vi "SLSC Convert EDS Property to SLSC Channel Path.vi"(0 "property":T3, 1 "GUID Get Properties Page":string, 2 "GUID Set Properties Page":string, 5 "Physical Channel":string, 12 "enums":T2[](array[typedef])) -> (3 "GUID Properties Page":string, 4 "name":string, 6 "Channel out":T4, 8 "SLSC Channel Path":string="Bool.LED1.NI.GreenBool", 10 "documentation-en":string, 13 "Cluster":T1, 14 "description-en":string)   [LabVIEW 2020, in "SLSC CD System Explorer.lvlib"]
uses:
  SLSC CD API/SLSC CD System Explorer/SLSC CD System Explorer.lvlib
  <vilib>/NI VeriStand/Custom Device API/Custom Device Channel.ctl
  <vilib>/NI VeriStand/Custom Device API/Custom Device Channel Type.ctl
  JSON parsing/property.ctl
  JSON parsing/enum.ctl
  <vilib>/NI VeriStand/Custom Device API/Custom Device API.lvlib
  SLSC CD API/SLSC CD Shared/SLSC CD Shared.lvlib
  SLSC UI API/SLSC Tree Control.lvlib
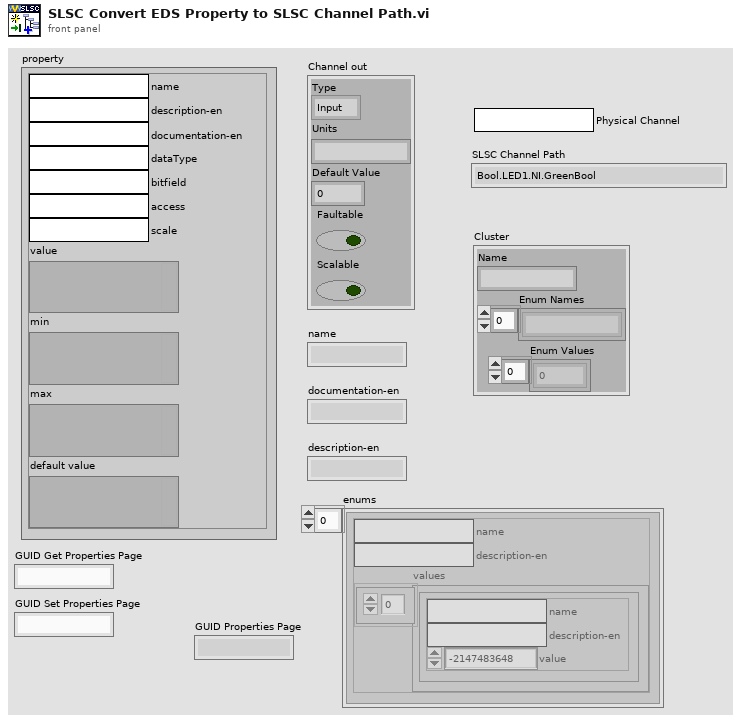
[diagram p1: front panel]
types:
  T1 = cluster{"Name":string, "Enum Names":string[], "Enum Values":i32[]}
  T2 = typedef "enum.ctl" = cluster{"name":string, "description-en":string, "values":cluster{"name":string, "description-en":string, "value":i32}[]}
  T3 = typedef "property.ctl" = cluster{"name":string, "description-en":string, "documentation-en":string, "dataType":string, "bitfield":string, "access":string, "scale":string, "value":variant, "min":variant, "max":variant, "default value":variant}
  T4 = typedef "Custom Device API.lvlib/Custom Device Channel.ctl" = cluster{"Type":T5, "Units":string, "Default Value":dbl, "Faultable":bool, "Scalable":bool}
  T5 = typedef "Custom Device API.lvlib/Custom Device Channel Type.ctl" = enum16{"Input", "Output"}
  T6 = cluster{"Name":string, "Enum Names":string[], "Enum Values":i32[]}[]
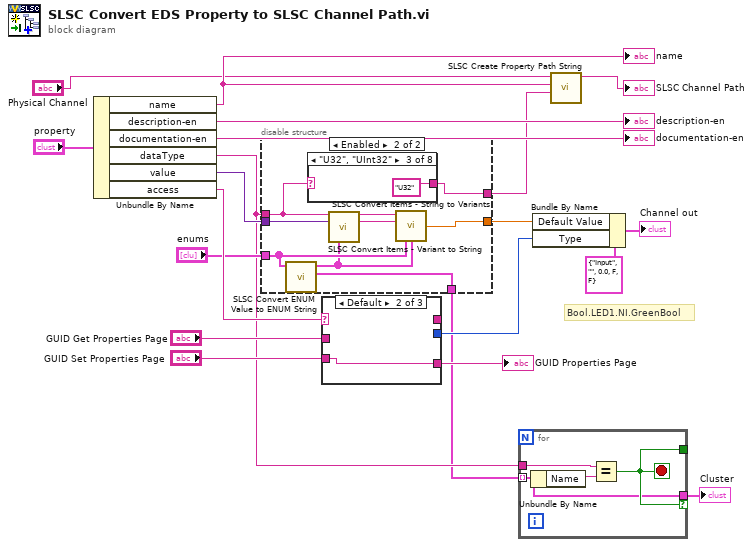
[diagram p0: block diagram]
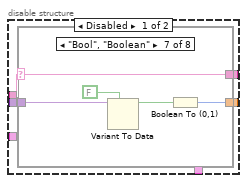
[diagram p2: hidden frame]
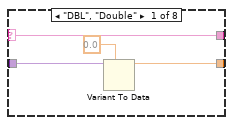
[diagram p3: hidden frame]
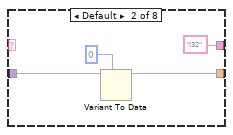
[diagram p4: hidden frame]
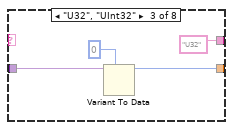
[diagram p5: hidden frame]
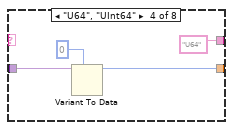
[diagram p6: hidden frame]
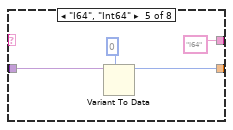
[diagram p7: hidden frame]
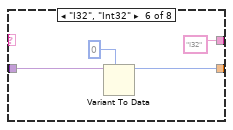
[diagram p8: hidden frame]
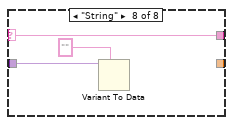
[diagram p9: hidden frame]
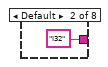
[diagram p11: hidden frame]
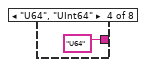
[diagram p12: hidden frame]
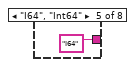
[diagram p13: hidden frame]
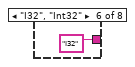
[diagram p14: hidden frame]
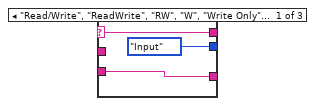
[diagram p17: hidden frame]
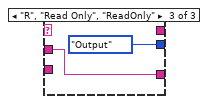
[diagram p18: hidden frame]
diagram:
  # "Bool.LED1.NI.GreenBool"
  n1 = Unbundle By Name("property") -> ("name"=w13:string, "description-en"=→"description-en":string, "documentation-en"=→"documentation-en":string, "dataType"=w3:string, "value"=w15:variant, "access"=w8:string)
  "name" <- w13
  n2 = disable-structure shown="Enabled" {
    disable-tunnel: w3 -> [w24 w59]
    disable-tunnel: w15 -> [w23 w63]
    disable-tunnel: [w22 w62] -> w14
    disable-tunnel: [w21 w58] -> w10
    disable-tunnel: "enums" -> [_ w61]
    disable-tunnel: [_ w57] -> w2
    frame Disabled {
      n3 = case shown="\"Bool\", \"Boolean\"" w24 {
        selector: w24 -> [w25 _ _ _ _ _ w49 w55]
        tunnel: w23 -> [w28 w30 w36 w40 w44 w48 w53 w56]
        tunnel: [w26 w29 w34 w38 w42 w46 w50 _] -> w22
        tunnel: [w25 "I32" "U32" "U64" "I64" "I32" w49 w55] -> w21
        frame "DBL", "Double" {
          n4 = Variant To Data(type=0.0, Variant=w28) -> (data=w26:dbl)  [unwired: 1 in, 1 out]
        }
        frame Default {
          n5 = Variant To Data(type=0, Variant=w30) -> (data=w29:i32)  [unwired: 1 in, 1 out]
        }
        frame "U32", "UInt32" {
          n6 = Variant To Data(type=u32 0, Variant=w36) -> (data=w34:u32)  [unwired: 1 in, 1 out]
        }
        frame "U64", "UInt64" {
          n7 = Variant To Data(type=u64 0, Variant=w40) -> (data=w38:u64)  [unwired: 1 in, 1 out]
        }
        frame "I64", "Int64" {
          n8 = Variant To Data(type=i64 0, Variant=w44) -> (data=w42:i64)  [unwired: 1 in, 1 out]
        }
        frame "I32", "Int32" {
          n9 = Variant To Data(type=0, Variant=w48) -> (data=w46:i32)  [unwired: 1 in, 1 out]
        }
        frame "Bool", "Boolean" {
          n10 = Variant To Data(type=FALSE, Variant=w53) -> (data=w51:bool)  [unwired: 1 in, 1 out]
          n11 = Boolean To (0,1)(Boolean=w51) -> (0, 1=w50:i16)
        }
        frame "String" {
          n12 = Variant To Data(type="", Variant=w56) -> ()  [unwired: 1 in, 2 out]
        }
      }
    }
    frame Enabled {
      n13 = call "SLSC Convert ENUM Value to ENUM String.vi"("Enums"=w61) -> ("Cluster Enums"=w57:T6, "String Enums"=w60:cluster{"name":string, "string enums":string}[])  [unwired: 9 in]
      n14 = case shown="\"U32\", \"UInt32\"" w59 {
        selector: w59 -> [w66 _ _ _ _ _ w72 w73]
        tunnel: [w66 "I32" "U32" "U64" "I64" "I32" w72 w73] -> w58
        frame "DBL", "Double" {
        }
        frame Default {
        }
        frame "U32", "UInt32" {
        }
        frame "U64", "UInt64" {
        }
        frame "I64", "Int64" {
        }
        frame "I32", "Int32" {
        }
        frame "Bool", "Boolean" {
        }
        frame "String" {
        }
      }
      n15 = call "SLSC Convert Items - Variant to String.vi"("Datatype"=w59, "value"=w63, "Enum string"=w60) -> ("Output data type"=w65:string, "string data value"=w64:string)  [unwired: 6 in, 5 out]
      n16 = call "SLSC Convert Items - String to Variants.vi"("Datatype"=w65, "Value"=w64, "enums"=w61, "string enums"=w60) -> ("Value (DBL)"=w62:dbl)  [unwired: 8 in, 3 out]
    }
  }
  n17 = case shown="Default" w8 {
    selector: w8 -> [w75 _ _]
    tunnel: [Custom_Device_Channel_Type."Input" ("Type") _ Custom_Device_Channel_Type."Output" ("Type")] -> w9
    tunnel: [w75 _ _] -> _
    tunnel: [w74 w77 w78] -> w7
    tunnel: "GUID Set Properties Page" -> [w74 w77 _]
    tunnel: "GUID Get Properties Page" -> [_ _ w78]
    frame "Read/Write", "ReadWrite", "RW", "W", "Write Only", "WriteOnly" {
    }
    frame Default {
    }
    frame "R", "Read Only", "ReadOnly" {
    }
  }
  "GUID Properties Page" <- w7
  n18 = for {
    tunnel: w2 -> [w80] mode=indexing
    tunnel: w3 -> [w82]
    tunnel: [w80] -> w1 if=w81
    tunnel: [w81] -> _
    stop <- w81 stop-if-true
    n19 = Unbundle By Name(w80) -> ("Name"=w83:string)
    n20 = Equal?(x=w82, y=w83) -> (x = y?=w81:bool)
  }
  "Cluster" <- w1
  n21 = Bundle By Name(cluster=T4 {"Type"=enum."Input", "Units"="", "Default Value"=0.0, "Faultable"=FALSE, "Scalable"=FALSE} ("Channel out"), "Default Value"=w14, "Type"=w9) -> (→"Channel out":T4)
  n22 = call "SLSC Create Property Path String.vi"("Datatype"=w10, "Property"=w13, "Physical Channel"="Physical Channel") -> ("SLSC Path String"=→"SLSC Channel Path":string)  [unwired: 8 in]
